vi "ep_Check Event Settings.vi"(8 "error in (no error)":errorcluster, 11 "events settings":T1={"swell threshold [%]"=110.0, "dip threshold [%]"=90.0, "interruption threshold [%]"=1.0, "hysteresis [%]"=2.0}) -> (0 "error out":errorcluster)   [LabVIEW 2014, in "NI_EP_Power Quality.lvlib"]
uses:
  <vilib>/addons/Electrical Power/PQ/NI_EP_Power Quality.lvlib
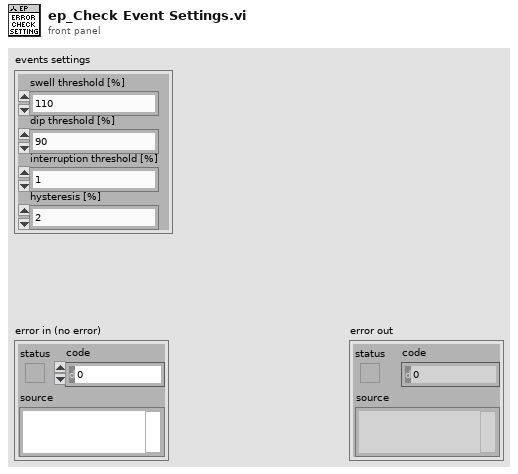
[diagram p1: front panel]
types:
  T1 = cluster{"swell threshold [%]":dbl, "dip threshold [%]":dbl, "interruption threshold [%]":dbl, "hysteresis [%]":dbl}
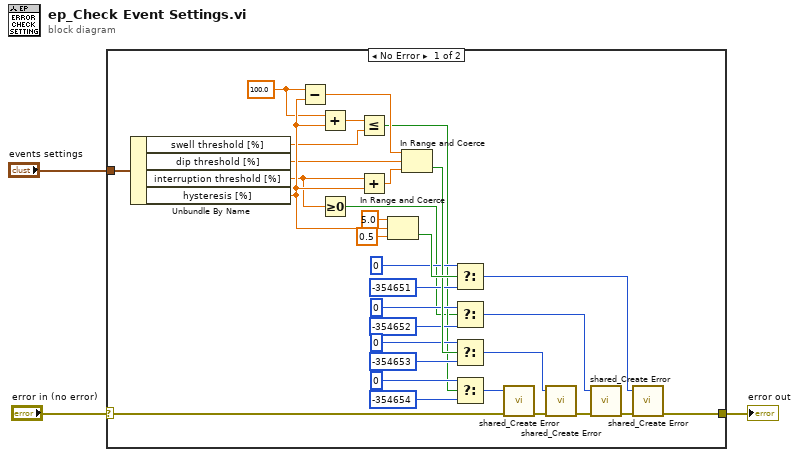
[diagram p0: block diagram]
diagram:
  n1 = case shown="No Error" "error in (no error)" {
    selector: "error in (no error)" -> [w4 w36]
    tunnel: "events settings" -> [w6 _]
    tunnel: [w5 w36] -> w1
    frame No Error {
      w26 = 100.0 ("x")
      n2 = Unbundle By Name(w6) -> ("swell threshold [%]"=w9:dbl, "dip threshold [%]"=w28:dbl, "interruption threshold [%]"=w8:dbl, "hysteresis [%]"=w29:dbl)
      n3 = Subtract(x=w26, y=w29) -> (x-y=w31:dbl)
      n4 = Add(x=w26, y=w29) -> (x+y=w32:dbl)
      n5 = Greater Or Equal To 0?(x=w8) -> (x >= 0?=w7:bool)
      n6 = Less Or Equal?(x=w32, y=w9) -> (x <= y?=w10:bool)
      n7 = Add(x=w8, y=w29) -> (x+y=w27:dbl)
      n8 = In Range and Coerce(upper limit=5.0, x=w29, lower limit=0.5) -> (In Range?=w33:bool)  [unwired: 1 out]
      n9 = In Range and Coerce(upper limit=w31, x=w28, lower limit=w27) -> (In Range?=w30:bool)  [unwired: 1 out]
      n10 = Select(t=0 ("error code (0)"), s=w33, f=-354651) -> (s? t:f=w11:i32)
      n11 = Select(t=0 ("error code (0)"), s=w7, f=-354652) -> (s? t:f=w15:i32)
      n12 = Select(t=0 ("error code (0)"), s=w30, f=-354653) -> (s? t:f=w17:i32)
      n13 = Select(t=0 ("error code (0)"), s=w10, f=-354654) -> (s? t:f=w20:i32)
      n14 = call <vilib>:"shared_Create Error.vi"("error in (no error)"=w4, "error code (0)"=w20) -> ("error out"=w18:errorcluster)  [unwired: 9 in]
      n15 = call <vilib>:"shared_Create Error.vi"("error in (no error)"=w18, "error code (0)"=w17) -> ("error out"=w14:errorcluster)  [unwired: 9 in]
      n16 = call <vilib>:"shared_Create Error.vi"("error in (no error)"=w14, "error code (0)"=w15) -> ("error out"=w13:errorcluster)  [unwired: 9 in]
      n17 = call <vilib>:"shared_Create Error.vi"("error in (no error)"=w13, "error code (0)"=w11) -> ("error out"=w5:errorcluster)  [unwired: 9 in]
    }
    frame Error {
    }
  }
  "error out" <- w1
